vi "Insert SubVI 2.vi"(0 "Sub Panel Ref":refnum<vi>, 1 "Label 1":string, 2 "Value 1":variant, 5 "VI Path":path, 7 "Label 3":string, 9 "Value 3":variant, 11 "error in (no error)":errorcluster, 12 "Label 2":string, 13 "Value 2":variant) -> (4 "vi reference":refnum<vi>, 15 "error out":errorcluster)   [LabVIEW 2020, in "2D Plot.lvclass"]
uses:
  <vilib>/Math Plots/2D Math Plots/2D Plot/2D Plot/2D Plot.lvclass
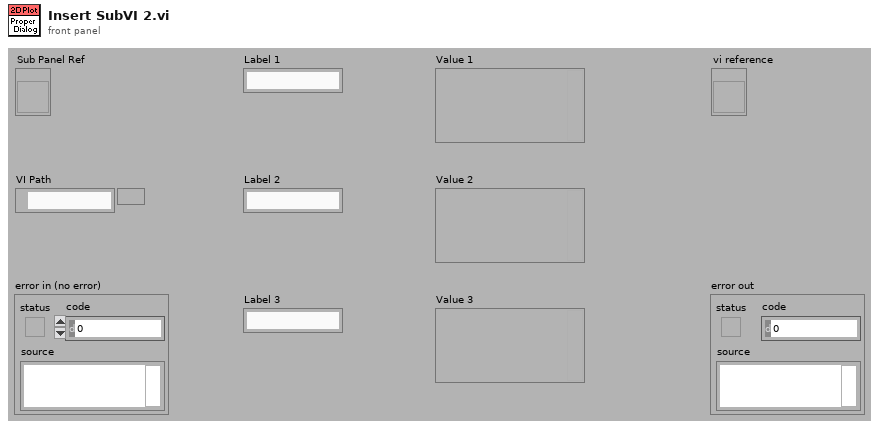
[diagram p1: front panel]
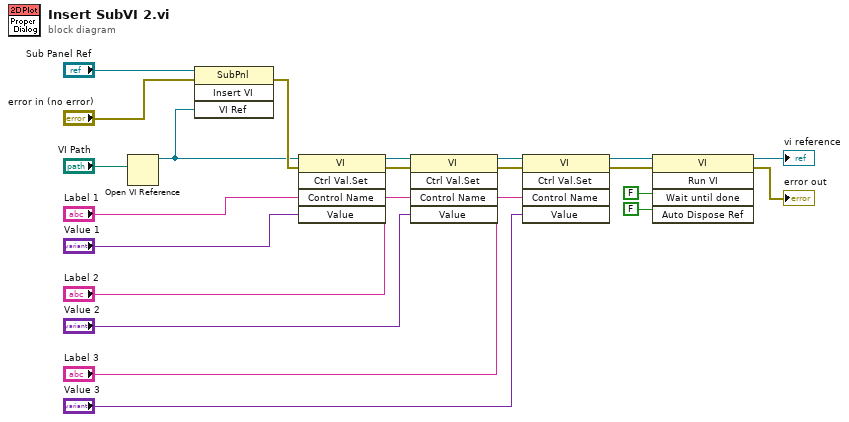
[diagram p0: block diagram]
diagram:
  n1 = Open VI Reference(vi path="VI Path") -> (vi reference=w15:refnum<vi>)  [unwired: 2 in, 4 out]
  n2 = invoke on="Invoke Node" class="SubPnl" method="Insert VI"(reference="Sub Panel Ref", error in="error in (no error)", "VI Ref"=w15) -> (error out=w16:errorcluster)  [unwired: 1 in, 3 out]
  n3 = invoke class="VI" method="Ctrl Val.Set"(reference=w15, error in=w16, "Control Name"="Label 1", "Value"="Value 1") -> (reference out=w19:refnum<vi>, error out=w21:errorcluster)  [unwired: 1 in, 3 out]
  n4 = invoke class="VI" method="Ctrl Val.Set"(reference=w19, error in=w21, "Control Name"="Label 2", "Value"="Value 2") -> (reference out=w6:refnum<vi>, error out=w5:errorcluster)  [unwired: 1 in, 3 out]
  n5 = invoke class="VI" method="Ctrl Val.Set"(reference=w6, error in=w5, "Control Name"="Label 3", "Value"="Value 3") -> (reference out=w4:refnum<vi>, error out=w3:errorcluster)  [unwired: 1 in, 3 out]
  n6 = invoke class="VI" method="Run VI"(reference=w4, error in=w3, "Wait until done"=FALSE ("Wait Until Done"), "Auto Dispose Ref"=FALSE ("Auto Dispose Reference")) -> (reference out=→"vi reference":refnum<vi>, error out=→"error out":errorcluster)  [unwired: 1 in, 3 out]
